vi "Insight_RW_Sweep_Profile_RollOff.vi"(7 "Parameter Type":enum16{"Value", "MAXimum", "MINimum", "DEFault"}(ring), 8 "error in (no error)":errorcluster, 9 "Mode (Read / Write)":enum8{"Write", "Read"}(ring), 10 "Roll-Off (dB)":dbl=3.0, 11 "telnet connection":T1) -> (0 "error out":errorcluster, 1 "response data":string, 2 "Roll-Off (dB)?":dbl, 3 "telnet  connection out":T1)   [LabVIEW 2011]
doc: "Insight Photonic Solutions\n\nThis VI sets or queries the decrease or roll-off, in dB relative to the peak, of a symmetric, non-flat wavelength vs. power profile. The best example is a Gaussian whose peak power is centered in the middle of the wavelength tuning range. As a further example, if the roll-off is set to 3dB, then the Full-Width at Half Maximum of the Gaussian is equal to the full wavelength tuning range.\n\nINPUT\nRoll-off - 0 to 10 dB\n\nOUTPUT\nresponse data - actual response string from the command or query\nRoll-off (dB) as parsed from the laser's response to the command\n\nINPUTS\n\nMode - Tells the VI whether the command is a Read or a Write. (Default = Read).\nParameter Type - Tells the VI whether the command should use a Value or a keyword MAXimum, MINimum or DEFault to set the parameter value. (Default = Value).\nRoll-Off (dB) - the roll-off of the power profile at the edge of the sweep. Assumes a symmetric profile, such as a Gaussian (Default = 10 dB).\nerror in - The standard LabView Error cluster. Use this to enforce sequentiality and error tracking.\n\nOUTPUTS\n\nresponse data - the complete response string from the laser\nRoll-Off (dB)? - the roll-off of the power profile at the edge of the sweep written to or read from the laser\nerror out - the standard error cluster. Reports errors in reading or writing to the laser, or passes through errors from before this VI.\n\n\nver 1.0 - original release\nver 3.4 - added parsing to handle versions 3.4 and later of Atlas\nver 3.5 - added ability to read/write Max, Min or Default keyword values"
uses:
  Telnet Session.ctl
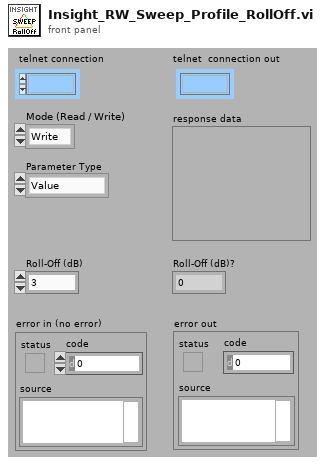
[diagram p1: front panel]
types:
  T1 = typedef "Telnet Session.ctl" = refnum<k1>
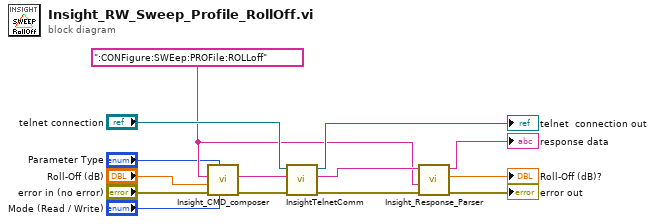
[diagram p0: block diagram]
diagram:
  w4 = ":CONFigure:SWEep:PROFile:ROLLoff" ("String")
  n1 = call "Insight_CMD_composer.vi"("Mode (Read / Write)"="Mode (Read / Write)", "Parameter Type"="Parameter Type", "error in (no error)"="error in (no error)", "Value"="Roll-Off (dB)", "CMD"=w4) -> ("error out"=w7:errorcluster, "Command String"=w5:string)  [unwired: 5 in]
  n2 = call "InsightTelnetComm.vi"("error in"=w7, "write buffer (\"\")"=w5, "telnet connection"="telnet connection") -> ("error out"=w12:errorcluster, "response data"=w10:string, "telnet  connection out"=→"telnet  connection out":T1)  [unwired: 4 in]
  n3 = call "Insight_Response_Parser.vi"("error in (no error)"=w12, "Command String"=w4, "Laser Response In"=w10) -> ("error out"=→"error out":errorcluster, "Value"=→"Roll-Off (dB)?":dbl, "Laser Response Out"=→"response data":string)  [unwired: 6 in]
